vi "Blur (Gaussian ARGB).vi"(5 "Sigma":T1, 6 "Border Type (Default: DEFAULT)":T3=enum."DEFAULT", 7 "Kernel Block Size":T2, 8 "error in (no error)":errorcluster, 10 "ARGB Gaussian Blur Result":T4, 11 "ARGB Image Source":T4) -> (0 "error out":errorcluster, 3 "ARGB Gaussian Blur Result (duplicate)":T4)   [LabVIEW 2020, in "g_ar_toolkit.image.lvlib"]
uses:
  g_ar_toolkit.image.lvlib
  ARGB Image.ctl
  Border Type.ctl
  Kernel Block Size.ctl
  g_ar_toolkit.common/Image Point (Float).ctl
  68bb216c-d3e3-4366-946f-f5b7f5c74ae7.vi
  g_ar_toolkit.common/Module Path.vi
  <vilib>/Utility/error.llb/Error Cluster From Error Code.vi
  g_ar_toolkit.common/g_ar_toolkit.common.lvlib
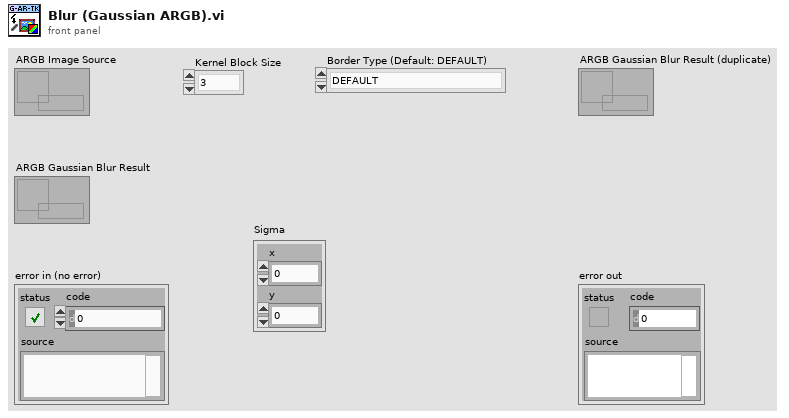
[diagram p1: front panel]
types:
  T1 = typedef "g_ar_toolkit.common.lvlib/Image Point (Float).ctl" = cluster{"x":dbl, "y":dbl}
  T2 = typedef "g_ar_toolkit.image.lvlib/Kernel Block Size.ctl" = enum16{"3", "5", "7", "9", "11", "13", "15", "17", "19", "21", "23", "25", "27", "29", "31", "33", "35", "37", "39", "41", "43", "45", "47", "49", "51", "53", "55", "57", "59", "61", "63", "65", "67", "69", "71", "73", "75", "77", "79", "81", "83", "85", "87", "89", "91", "93", "95", "97", "99", "101", "103", "105", "107", "109", "111", "113", "115", "117", "119", "121", "123", "125", "127", "129", "131", "133", "135", "137", "139", "141", "143", "145", "147", "149", "151", "153", "155", "157", "159", "161", "163", "165", "167", "169", "171", "173", "175", "177", "179", "181", "183", "185", "187", "189", "191", "193", "195", "197", "199", "201", "203", "205", "207", "209", "211", "213", "215", "217", "219", "221", "223", "225", "227", "229", "231", "233", "235", "237", "239", "241", "243", "245", "247", "249", "251", "253", "255", "257", "259", "261", "263", "265", "267", "269", "271", "273", "275", "277", "279", "281", "283", "285", "287", "289", "291", "293", "295", "297", "299", "301", "303", "305", "307", "309", "311", "313", "315", "317", "319", "321", "323", "325", "327", "329", "331", "333", "335", "337", "339", "341", "343", "345", "347", "349", "351", "353", "355", "357"}
  T3 = typedef "g_ar_toolkit.image.lvlib/Border Type.ctl" = enum8{"CONSTANT", "REPLICATE", "REFLECT", "WRAP", "TRANSPARENT", "DEFAULT", "ISOLATED"}
  T4 = typedef "g_ar_toolkit.image.lvlib/ARGB Image.ctl" = refnum<data-value>
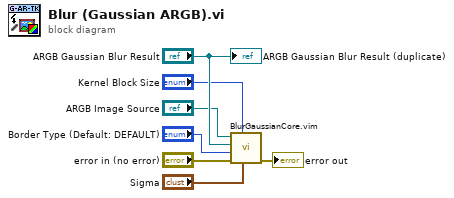
[diagram p0: block diagram]
diagram:
  n1 = call "BlurGaussianCore.vim"("Sigma"="Sigma", "Kernel Block Size"="Kernel Block Size", "error in (no error)"="error in (no error)", "Border Type"="Border Type (Default: DEFAULT)", "Gaussian Blur Result"="ARGB Gaussian Blur Result", "Data Value Reference in"="ARGB Image Source") -> ("error out"=→"error out":errorcluster)  [unwired: 5 in]
  "ARGB Gaussian Blur Result (duplicate)" <- "ARGB Gaussian Blur Result"
